vi "Station Wise_summary.vi"(0 "index":i32, 1 "Station ID":string, 3 "error in (no error)":errorcluster, 4 "Station Name":string) -> (6 "S":bool, 7 "M":bool, 9 "error out":errorcluster)   [LabVIEW 2017]
uses:
  <vilib>/addons/database/Connection.llb/DB Tools Open Connec (Path).vi
  Globle/Current date.vi
  <vilib>/addons/database/NI_Database_API.lvlib
panel:
  out "Station Name":string
  in  "Cancel Button":bool
  out "G Ack 2":bool
  out "GL 2":bool
  out "Duration P":dbl format="%<%M:%S>t"
  out "Duration Q":dbl format="%<%M:%S>t"
  out "Duration M":dbl format="%<%M:%S>t"
  out "Duration L":dbl format="%<%M:%S>t"
  out "Duration GL":dbl format="%<%M:%S>t"
  out "COUNT P":i32
  out "COUNT  Q":i32
  out "COUNT  M":i32
  out "COUNT  Mat":i32
  out "P Ack":bool
  out "Q Ack":bool
  out "M Ack":bool
  out "L Ack":bool
  out "G Ack":bool
  out "SS":bool
  out "Q":bool
  out "M":bool
  out "COUNT Safety":i32
  out "P Duration Min":dbl format="%<%M:%S>t"
  out "Q Duration Min":dbl format="%<%M:%S>t"
  out "M Duration Min":dbl format="%<%M:%S>t"
  out "L Duration Min":dbl format="%<%M:%S>t"
  out "GL Duration min":dbl format="%<%M:%S>t"
  out "P Counter":i32
  out "Q Counter":i32
  out "M Counter":i32
  out "Mat Counter":i32
  out "Safety Counter":i32
  # "Station Wise Live Breakdown Status"
  # "Safety"
  # "Material"
  # "Maintenance"
  # "Quality"
  # "Startup/Setup"
  # "Stakeholder"
  # "Count"
  # "Duration"
  # "Station"
  # "Breakdown Name"
  # "Safety"
  # "Min"
  # "Breakdown"
  # "Material"
  # "Min"
  # "Acknowledgement"
  # "Maintenance"
  # "Min"
  # "Total Count"
  # "Quality"
  # "Min"
  # "Total Duration (Min)"
  # "Startup/Setup"
  # "Min"
  # "Designed And Developed By - Infinity Automation Systems Pvt. Ltd."
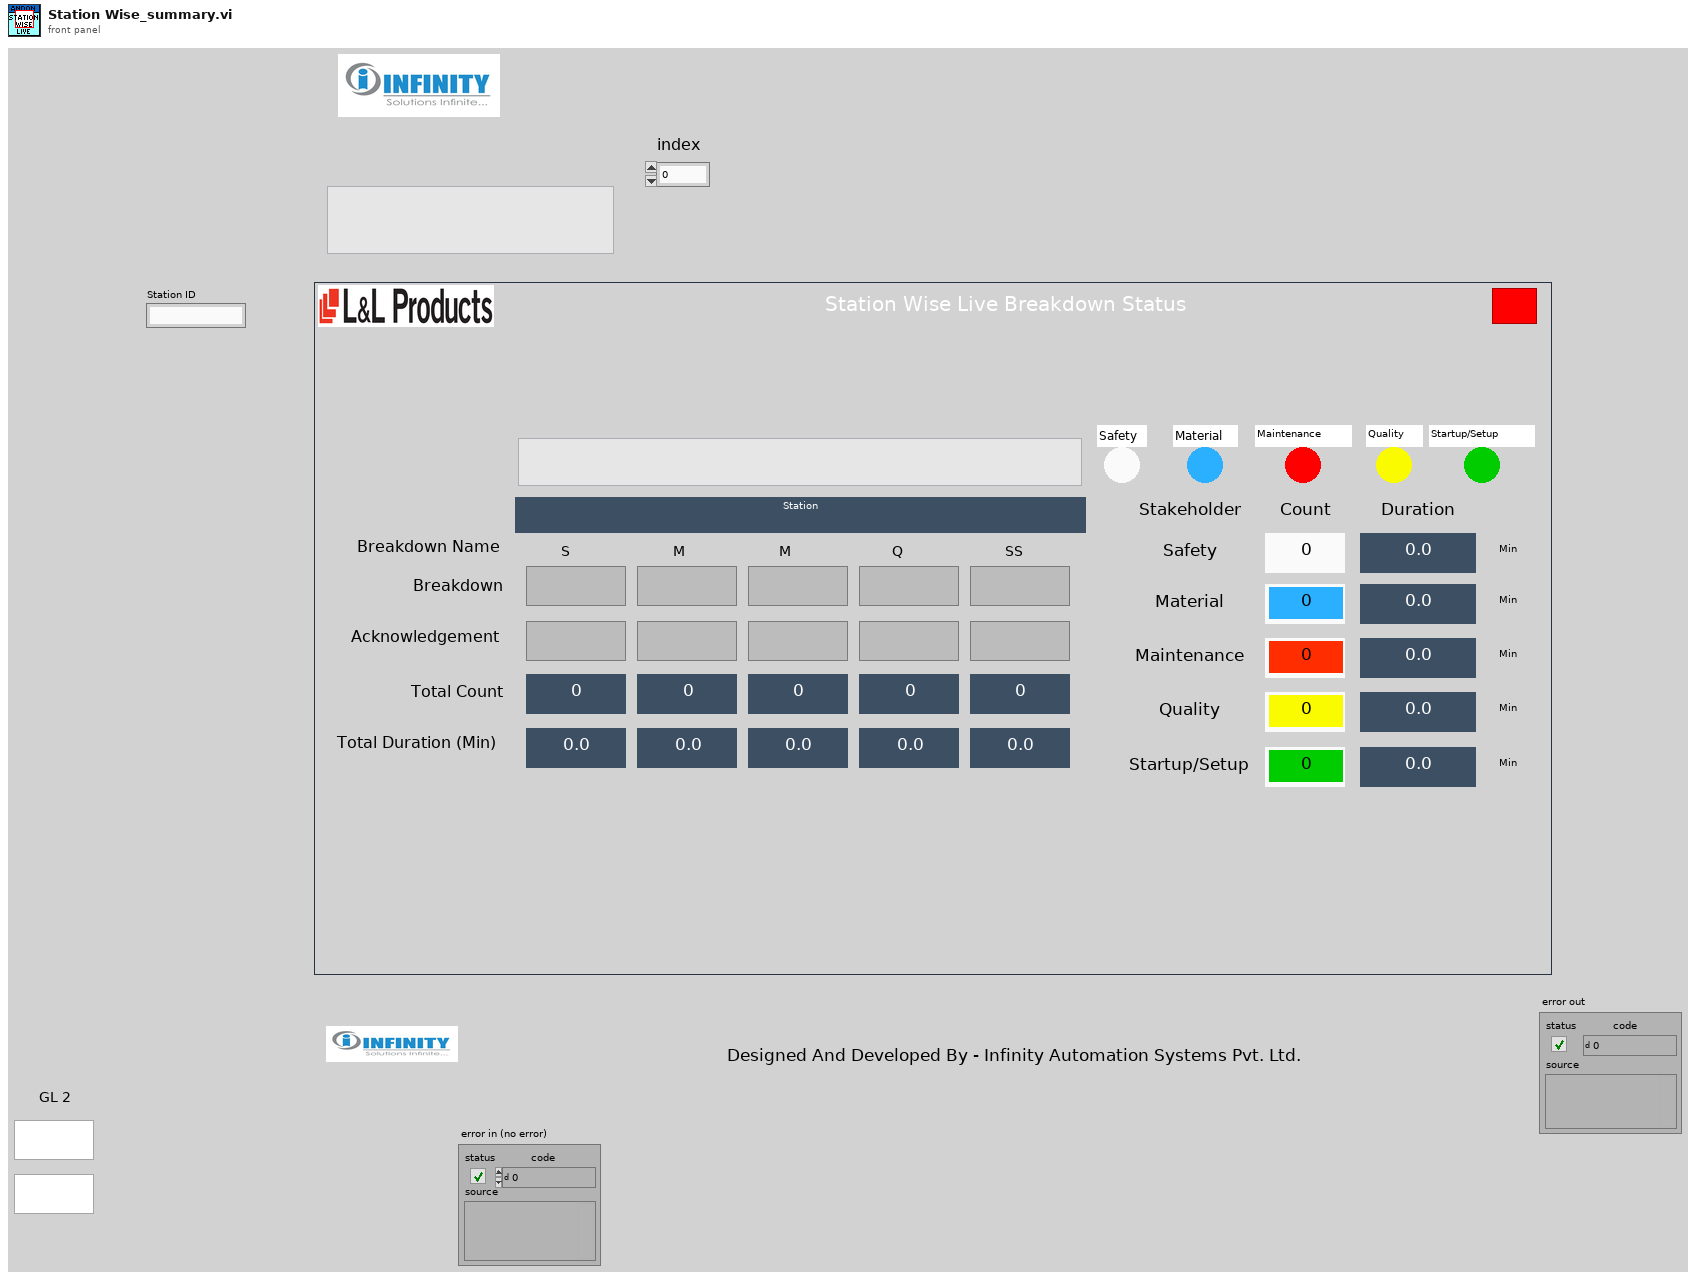
[diagram p1: front panel]
types:
  T1 = typedef "NI_Database_API.lvlib/Conn ObjectReference.ctl" = refnum<k1>
  T2 = enum32{"invalid app kind", "Development System", "Run Time System", "Student Edition", "Embedded LabVIEW", "Evaluation", "Custom"}
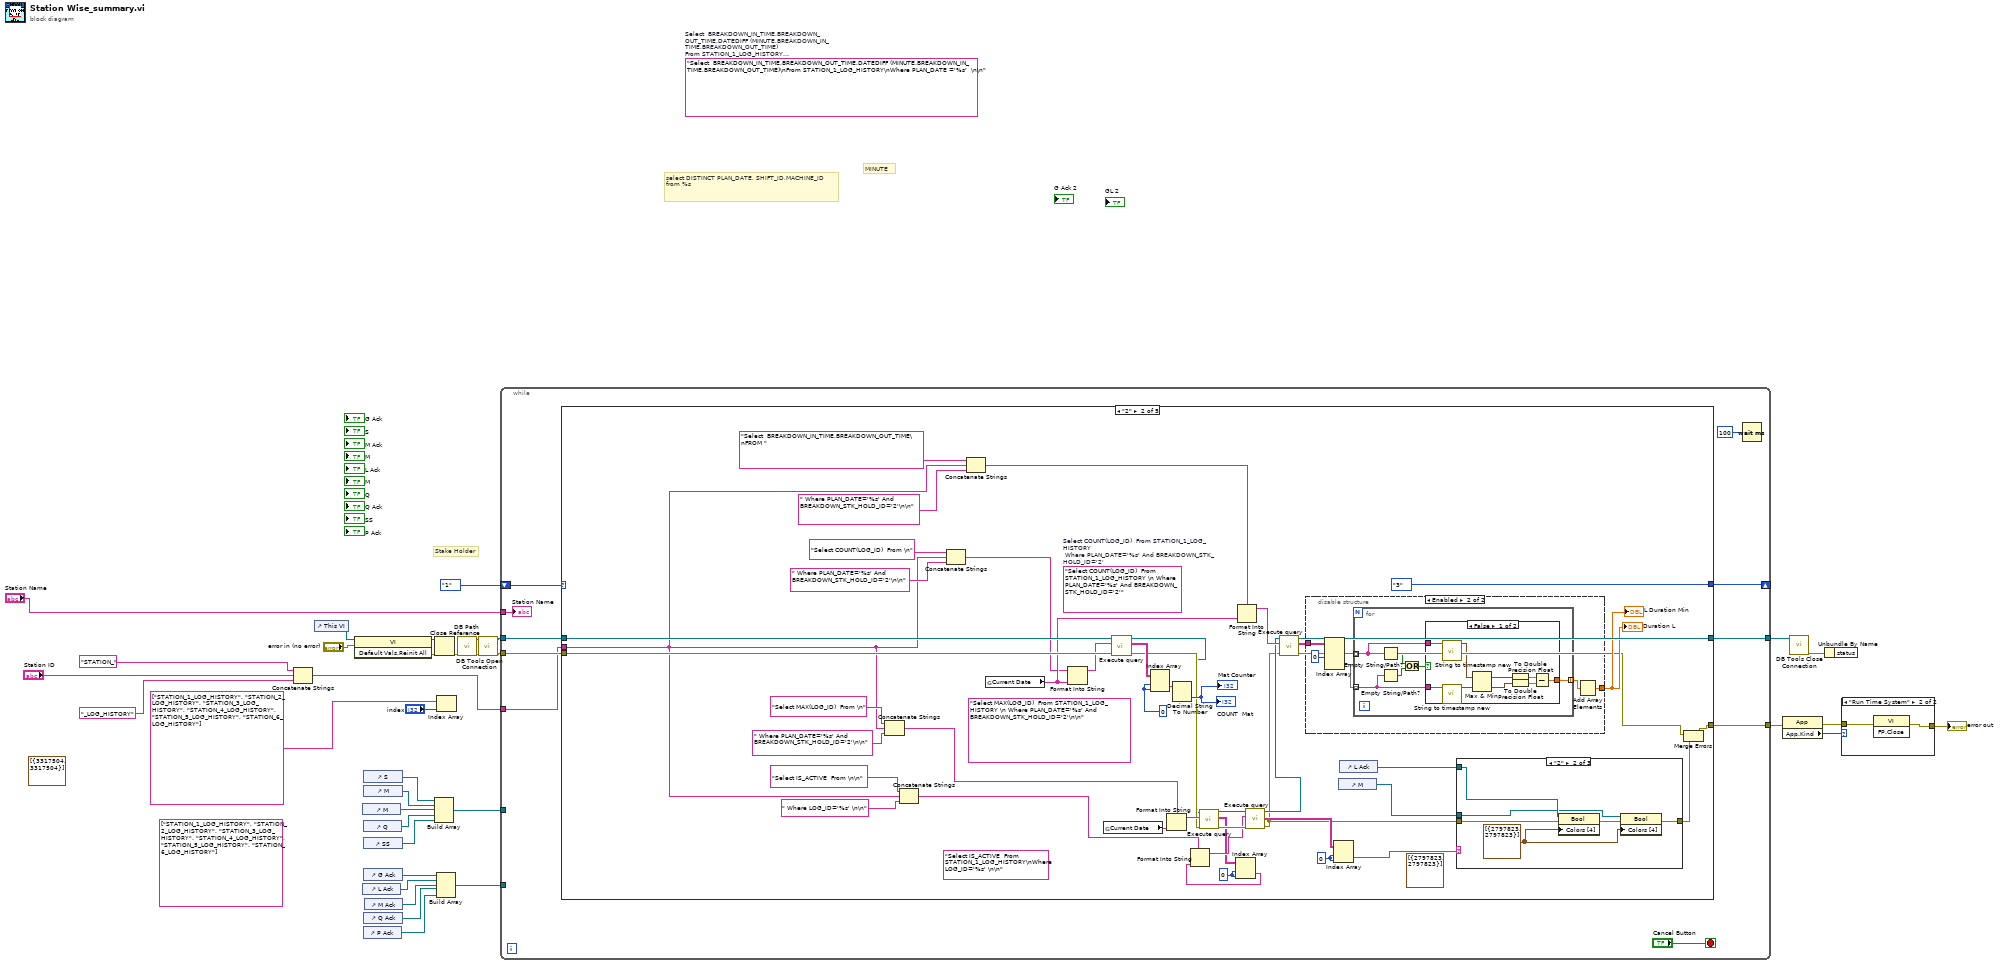
[diagram p0: block diagram]
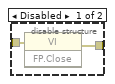
[diagram p3: hidden frame]
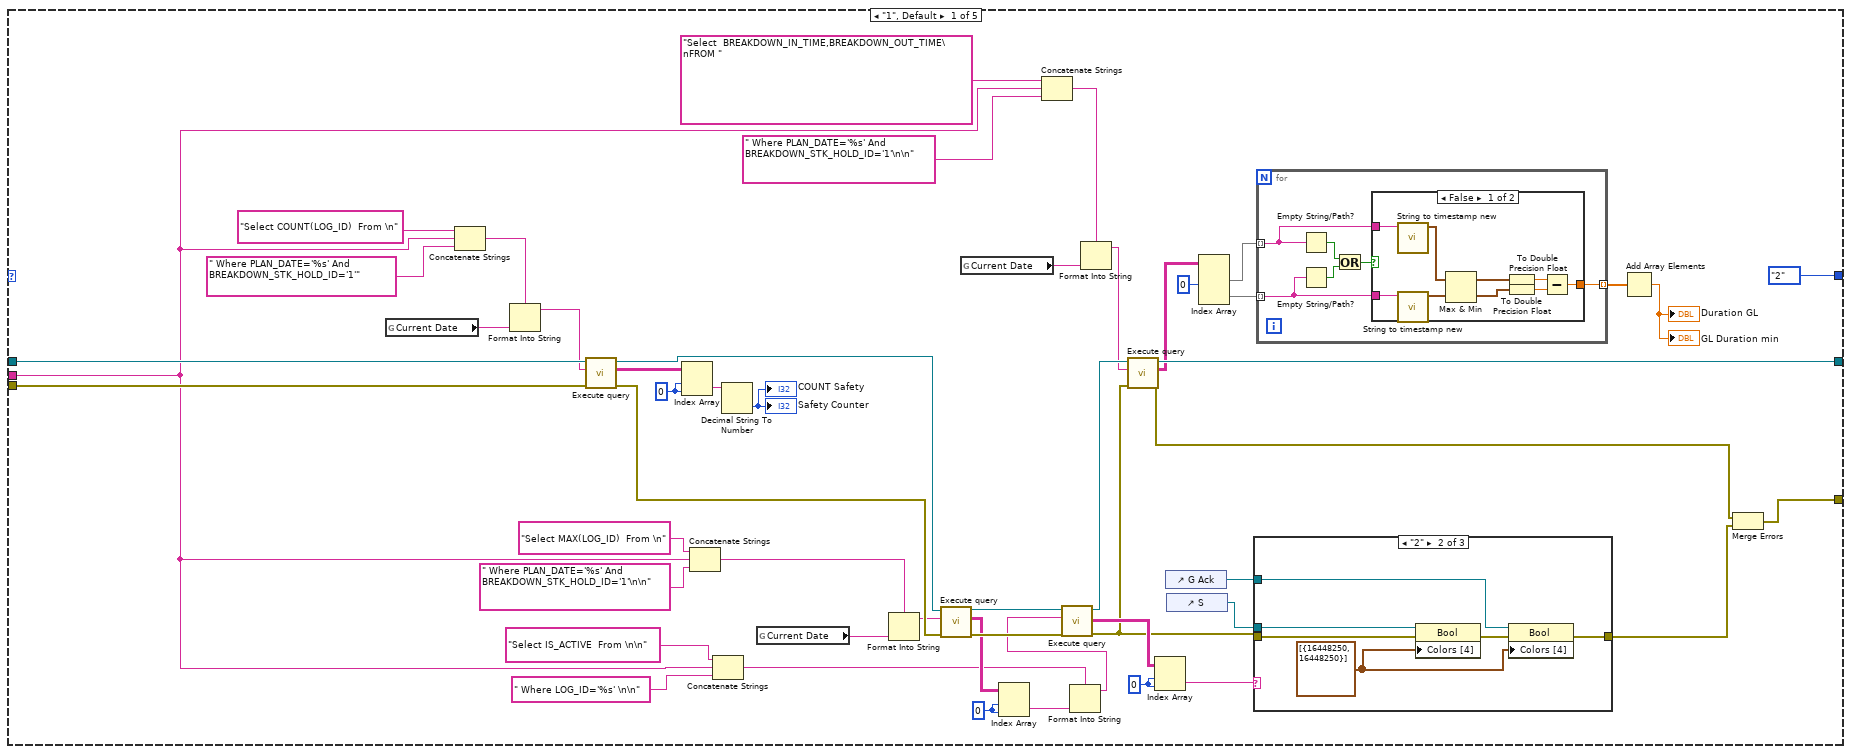
[diagram p4: hidden frame]
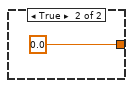
[diagram p5: hidden frame]
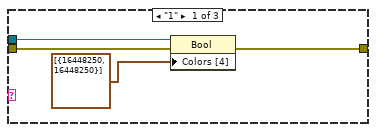
[diagram p6: hidden frame]
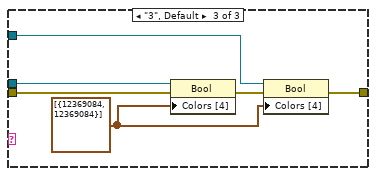
[diagram p7: hidden frame]
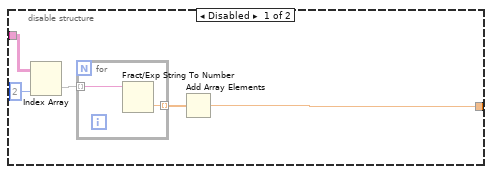
[diagram p8: hidden frame]
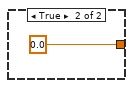
[diagram p9: hidden frame]
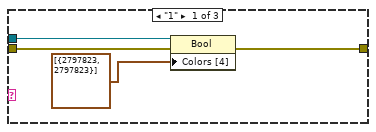
[diagram p10: hidden frame]
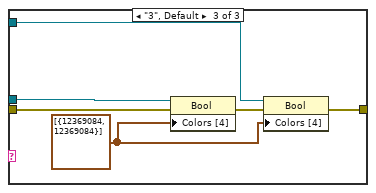
[diagram p11: hidden frame]
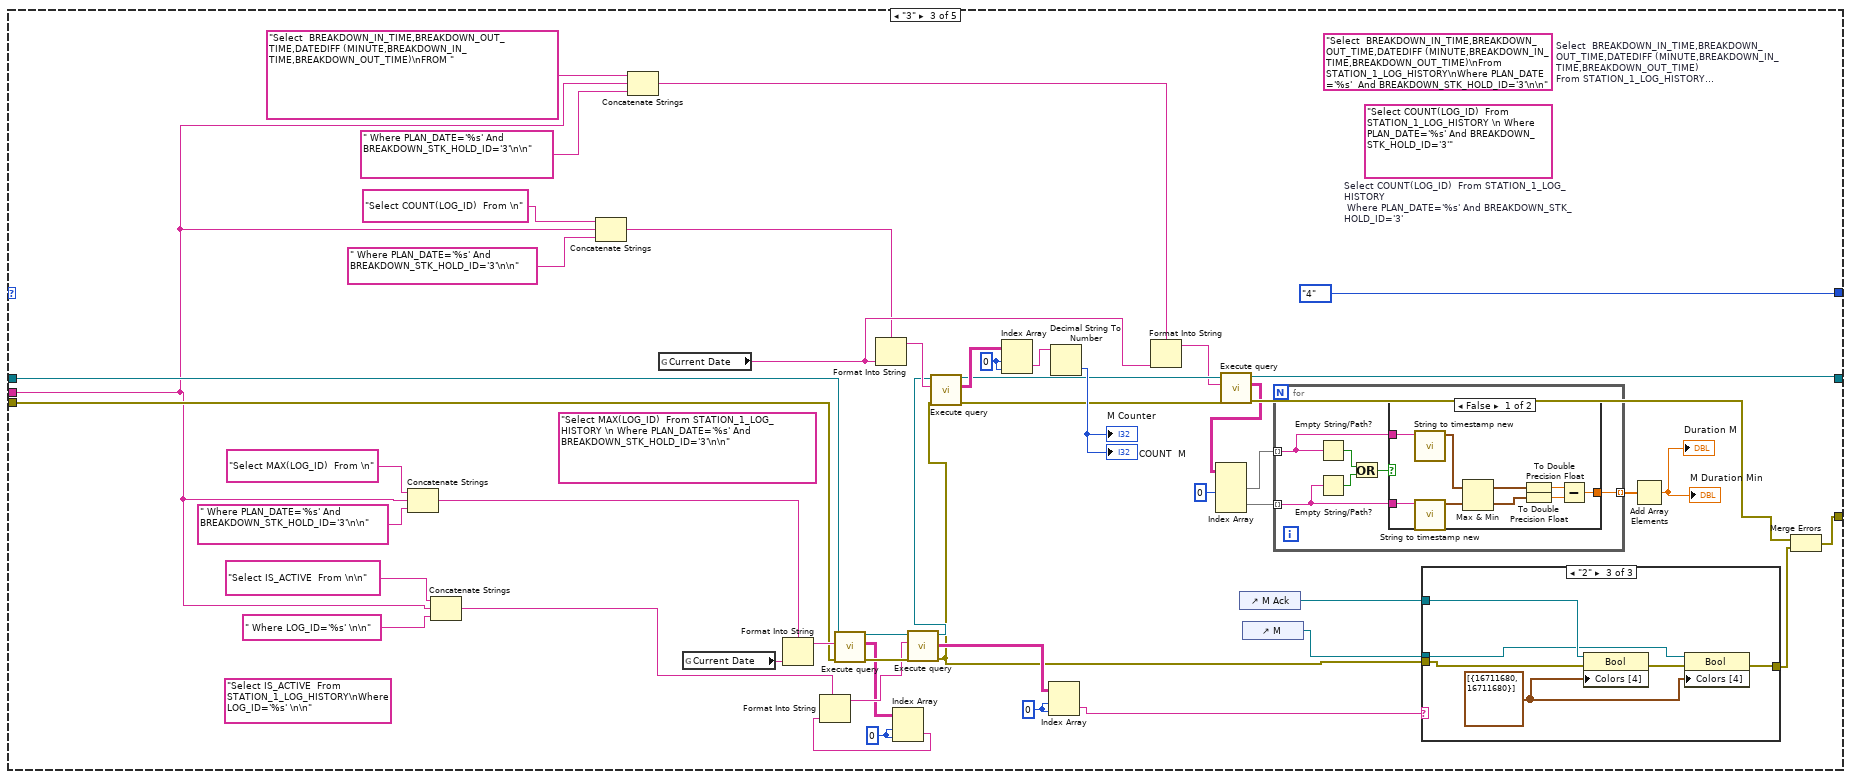
[diagram p12: hidden frame]
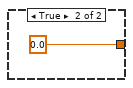
[diagram p13: hidden frame]
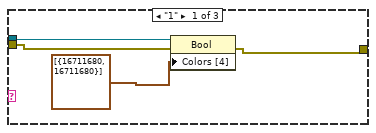
[diagram p14: hidden frame]
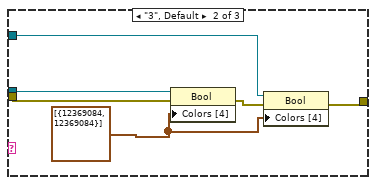
[diagram p15: hidden frame]
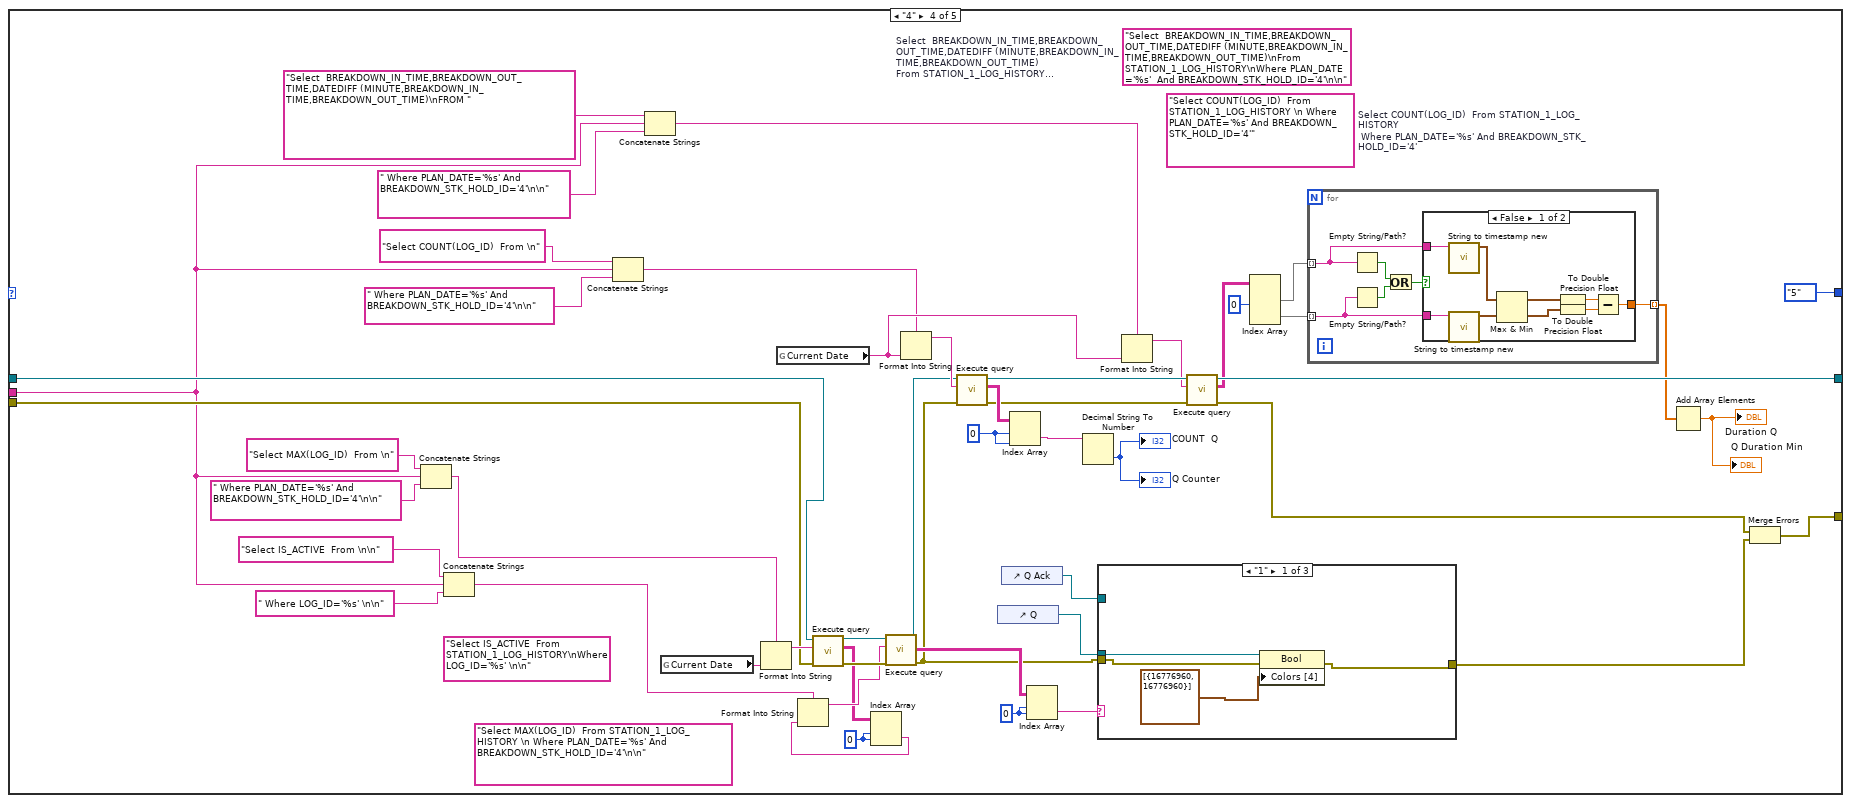
[diagram p16: hidden frame]
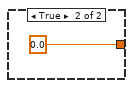
[diagram p17: hidden frame]
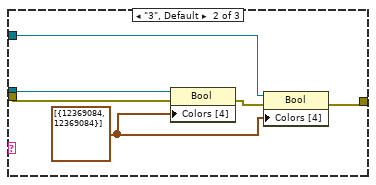
[diagram p18: hidden frame]
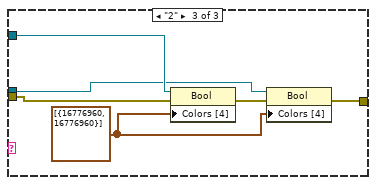
[diagram p19: hidden frame]
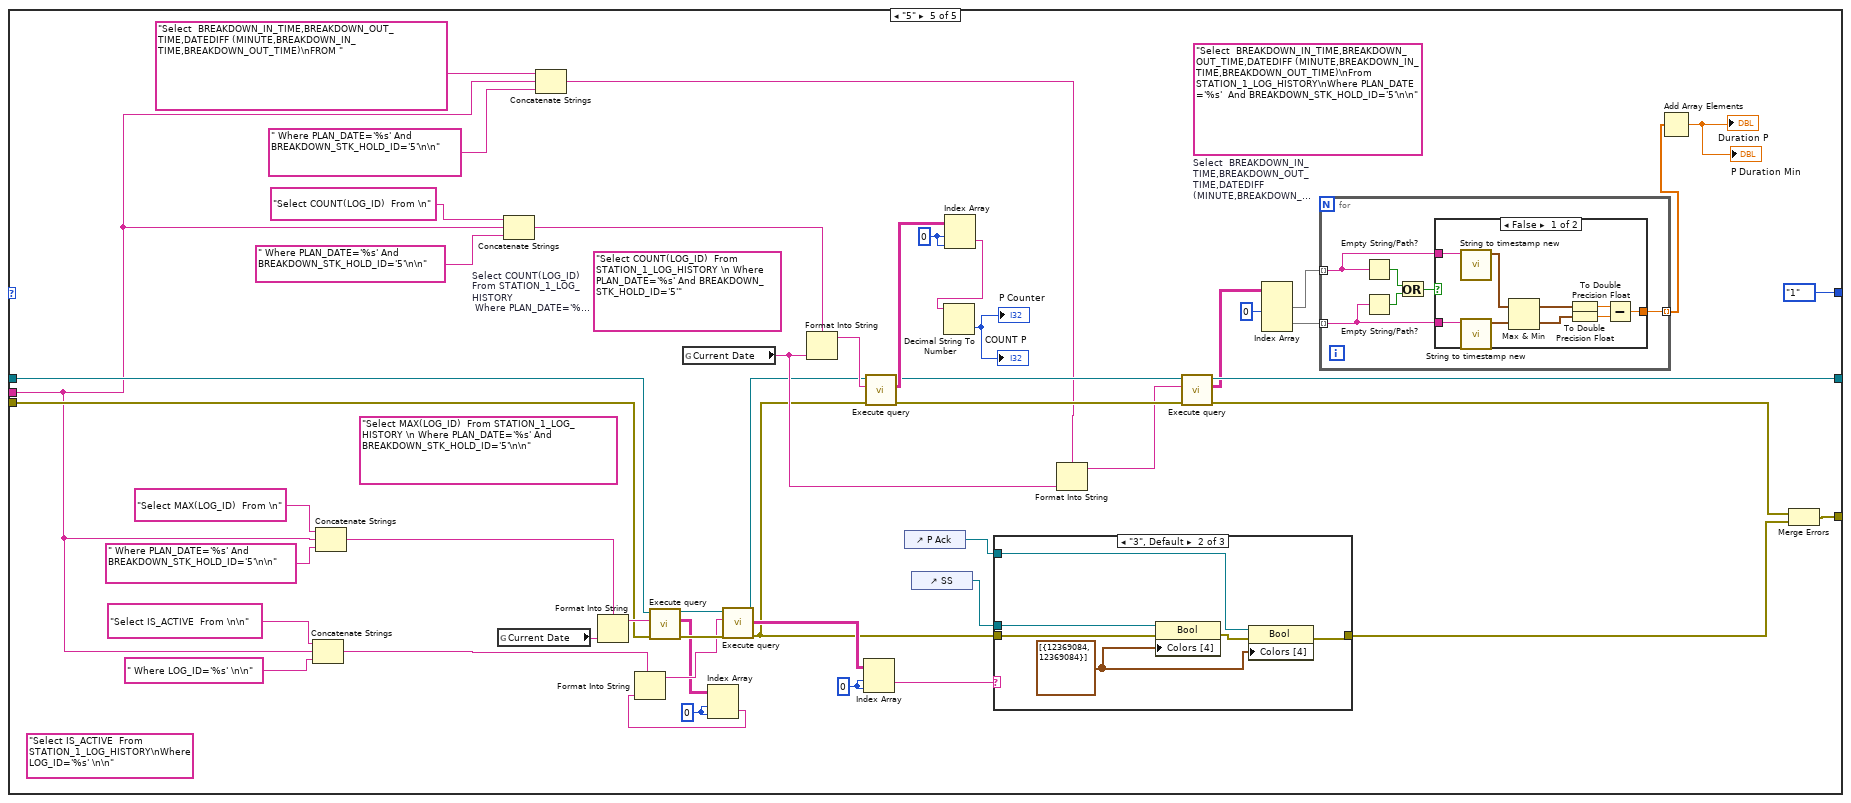
[diagram p20: hidden frame]
diagram:
  (unwired) string[] ["STATION_1_LOG_HISTORY", "STATION_2_LOG_HISTORY", "STATION_3_LOG_HISTORY", "STATION_4_LOG_HISTORY", "STATION_5_LOG_HISTORY", "STATION_6_LOG_HISTORY"]
  (unwired) "Select  BREAKDOWN_IN_TIME,BREAKDOWN_OUT_TIME,DATEDIFF (MINUTE,BREAKDOWN_IN_TIME,BREAKDOWN_OUT_TIME)\nFrom STATION_1_LOG_HISTORY\nWhere PLAN_DATE ='%s'  \n\n"  # Select  BREAKDOWN_IN_TIME,BREAKDOWN_OUT_TIME,DATEDIFF (MINUTE,BREAKDOWN_IN_TIME,BREAKDOWN_OUT_TIME) From STATION_1_LOG_HISTORY Where PLAN_DATE ='%s'
  (unwired) cluster{u32, u32}[] [{3317504, 3317504}] ("Colors [4]")
  # "Stake Holder"
  # "MINUTE"
  # "select DISTINCT PLAN_DATE, SHIFT_ID,MACHINE_ID\nfrom %s"
  n1 = Concatenate Strings("STATION_", "Station ID", "_LOG_HISTORY") -> (w5:string)
  n2 = control-ref of="This VI"() -> (w35:refnum<vi>)
  n3 = invoke class="VI" method="Default Vals.Reinit All"(reference=w35, error in="error in (no error)") -> (reference out=w33:refnum<vi>, error out=w34:errorcluster)  [unwired: 1 in, 1 out]
  n4 = control-ref of="M"() -> (w21:refnum<vi>)
  n5 = control-ref of="L Ack"() -> (w17:refnum<vi>)
  n6 = control-ref of="Q"() -> (w20:refnum<vi>)
  n7 = control-ref of="P Ack"() -> (w14:refnum<vi>)
  n8 = control-ref of="S"() -> (w23:refnum<vi>)
  n9 = control-ref of="M"() -> (w22:refnum<vi>)
  n10 = control-ref of="SS"() -> (w19:refnum<vi>)
  n11 = control-ref of="G Ack"() -> (w18:refnum<vi>)
  n12 = control-ref of="Q Ack"() -> (w15:refnum<vi>)
  n13 = control-ref of="M Ack"() -> (w16:refnum<vi>)
  n14 = Build Array(w23, w22, w21, w20, w19) -> (w13:refnum<vi>[])
  n15 = Close Reference(reference=w33, error in (no error)=w34) -> (error out=w29:errorcluster)
  n16 = Build Array(w18, w17, w16, w15, w14) -> (w12:refnum<vi>[])
  n17 = Index Array(array=string[] ["STATION_1_LOG_HISTORY", "STATION_2_LOG_HISTORY", "STATION_3_LOG_HISTORY", "STATION_4_LOG_HISTORY", "STATION_5_LOG_HISTORY", "STATION_6_LOG_HISTORY"], index="index") -> ()  [unwired: 1 out]
  n18 = call "DB Path.vi"("error in"=w29) -> ("error out"=w28:errorcluster, "DB Path"=w27:path)  [unwired: 9 in]
  n19 = call-poly <vilib>:"DB Tools Open Connection.vi"("error in (no error)"=w28, "connection information"=w27) -> ("error out"=w9:errorcluster, "connection reference"=w26:T1)  [unwired: 6 in]
  n20 = while {
    tunnel: w9 -> [w40]
    tunnel: [w45] -> w30
    tunnel: w26 -> [w41]
    tunnel: w5 -> [w39]
    shift-right: [w43] -> _
    shift-left: enum16{"1", "2", "3", "4", "5"}."1" -> [w44]
    tunnel: [w42] -> w8
    tunnel: w13 -> [_]
    tunnel: w12 -> [_]
    tunnel: "Station Name" -> [w36]
    stop <- "Cancel Button" stop-if-true
    n21 = case shown="\"2\"" w44 {
      tunnel: w40 -> [w90 w172 w244 w328 w411]
      tunnel: w41 -> [w96 w171 w243 w327 w410]
      tunnel: w39 -> [w58 w130 w226 w307 w392]
      tunnel: [w72 w145 w255 w320 w404] -> w45
      tunnel: [enum16{"1", "2", "3", "4", "5"}."2" enum16{"1", "2", "3", "4", "5"}."3" enum16{"1", "2", "3", "4", "5"}."4" enum16{"1", "2", "3", "4", "5"}."5" enum16{"1", "2", "3", "4", "5"}."1"] -> w43
      tunnel: [w91 w166 w261 w343 w425] -> w42
      frame "1", Default {
        w76 = 0 ("index (row)")
        w79 = 0 ("index (row)")
        w93 = 0 ("index (row)")
        n22 = global read "Current date.vi" "Current Date"() -> (w89:string)
        n23 = Concatenate Strings("Select COUNT(LOG_ID)  From \n", w58, " Where PLAN_DATE='%s' And BREAKDOWN_STK_HOLD_ID='1'") -> (w53:string)
        n24 = Format Into String(format string=w53, w89) -> (resulting string=w63:string)  [unwired: 2 in, 1 out]
        n25 = call "Execute query.vi"("error in (no error)"=w90, "String"=w63, "connection reference"=w96) -> ("error out"=w86:errorcluster, "Table"=w88:string[][], "connection reference 2"=w84:T1)  [unwired: 3 in, 3 out]
        n26 = Index Array(array=w88, index (row)=w93, index (col)=w93) -> (element=w92:string)
        n27 = Concatenate Strings("Select MAX(LOG_ID)  From \n", w58, " Where PLAN_DATE='%s' And BREAKDOWN_STK_HOLD_ID='1'\n\n") -> (w52:string)
        n28 = Concatenate Strings("Select IS_ACTIVE  From \n\n", w58, " Where LOG_ID='%s' \n\n") -> (w55:string)
        n29 = Decimal String To Number(string=w92) -> (number=→"Safety Counter" →"COUNT Safety":i32)  [unwired: 2 in, 1 out]
        n30 = global read "Current date.vi" "Current Date"() -> (w87:string)
        n31 = Format Into String(format string=w52, w87) -> (resulting string=w85:string)  [unwired: 2 in, 1 out]
        n32 = call "Execute query.vi"("error in (no error)"=w86, "String"=w85, "connection reference"=w84) -> ("error out"=w83:errorcluster, "Table"=w78:string[][], "connection reference 2"=w82:T1)  [unwired: 3 in, 3 out]
        n33 = global read "Current date.vi" "Current Date"() -> (w65:string)
        n34 = Index Array(array=w78, index (row)=w79, index (col)=w79) -> (element=w77:string)
        n35 = Concatenate Strings("Select  BREAKDOWN_IN_TIME,BREAKDOWN_OUT_TIME\nFROM " ("SQL query"), w58, " Where PLAN_DATE='%s' And BREAKDOWN_STK_HOLD_ID='1'\n\n") -> (w54:string)
        n36 = Format Into String(format string=w55, w77) -> (resulting string=w80:string)  [unwired: 2 in, 1 out]
        n37 = call "Execute query.vi"("error in (no error)"=w83, "String"=w80, "connection reference"=w82) -> ("error out"=w74:errorcluster, "Table"=w75:string[][], "connection reference 2"=w81:T1)  [unwired: 3 in, 3 out]
        n38 = Format Into String(format string=w54, w65) -> (resulting string=w64:string)  [unwired: 2 in, 1 out]
        n39 = call "Execute query.vi"("error in (no error)"=w74, "String"=w64, "connection reference"=w81) -> ("error out"=w73:errorcluster, "Table"=w51:string[][], "connection reference 2"=w91:T1)  [unwired: 3 in, 3 out]
        n40 = Index Array(array=w75, index (row)=w76, index (col)=w76) -> (element=w68:string)
        n41 = control-ref of="G Ack"() -> (w69:refnum<vi>)
        n42 = control-ref of="S"() -> (w70:refnum<vi>)
        n43 = Index Array(array=w51, index (col) #1=0 ("disabled index (col)")) -> (element #1=w49:string[], element #2=w48:string[])  [unwired: 3 in]
        n44 = case shown="\"2\"" w68 {
          tunnel: w74 -> [w116 w122 w128]
          tunnel: [w114 w119 w125] -> w71
          tunnel: w70 -> [w113 w118 w124]
          tunnel: w69 -> [_ w117 w123]
          frame "1" {
            n45 = property class="Bool"(reference=w113, error in=w116, "Colors [4]"=cluster{u32, u32}[] [{16448250, 16448250}]) -> (error out=w114:errorcluster)  [unwired: 1 out]
          }
          frame "2" {
            w120 = cluster{u32, u32}[] [{16448250, 16448250}] ("Colors [4]")
            n46 = property class="Bool"(reference=w118, error in=w122, "Colors [4]"=w120) -> (error out=w121:errorcluster)  [unwired: 1 out]
            n47 = property class="Bool"(reference=w117, error in=w121, "Colors [4]"=w120) -> (error out=w119:errorcluster)  [unwired: 1 out]
          }
          frame "3", Default {
            w126 = cluster{u32, u32}[] [{12369084, 12369084}] ("Colors [4]")
            n48 = property class="Bool"(reference=w124, error in=w128, "Colors [4]"=w126) -> (error out=w127:errorcluster)  [unwired: 1 out]
            n49 = property class="Bool"(reference=w123, error in=w127, "Colors [4]"=w126) -> (error out=w125:errorcluster)  [unwired: 1 out]
          }
        }
        n50 = for {
          tunnel: w49 -> [w98] mode=indexing
          tunnel: w48 -> [w99] mode=indexing
          tunnel: [w97] -> w47 mode=indexing
          n51 = Empty String/Path?(string/path=w98) -> (empty?=w101:bool)
          n52 = Empty String/Path?(string/path=w99) -> (empty?=w102:bool)
          n53 = Or(x=w101, y=w102) -> (x .or. y?=w100:bool)
          n54 = case shown="False" w100 {
            tunnel: [w105 0.0] -> w97
            tunnel: w98 -> [w104 _]
            tunnel: w99 -> [w103 _]
            frame False {
              n55 = call "String to timestamp new.vi"("String Timestamp"=w104) -> ("Timestamp"=w107:timestamp)  [unwired: 10 in]
              n56 = call "String to timestamp new.vi"("String Timestamp"=w103) -> ("Timestamp"=w106:timestamp)  [unwired: 10 in]
              n57 = Max & Min(x=w107, y=w106) -> (max(x,y)=w111:timestamp, min(x,y)=w110:timestamp)
              n58 = To Double Precision Float(number=w111) -> (double precision float=w109:dbl)
              n59 = To Double Precision Float(number=w110) -> (double precision float=w108:dbl)
              n60 = Subtract(x=w109, y=w108) -> (x-y=w105:dbl)
            }
            frame True {
            }
          }
        }
        n61 = Add Array Elements(numeric array=w47) -> (sum=→"GL Duration min" →"Duration GL":dbl)
        n62 = Merge Errors(w73, w71) -> (w72:errorcluster)
      }
      frame "2" {
        (unwired) cluster{u32, u32}[] [{2797823, 2797823}] ("Colors [4]")
        w154 = 0 ("index (row)")
        w157 = 0 ("index (row)")
        (unwired) "Select IS_ACTIVE  From STATION_1_LOG_HISTORY\nWhere LOG_ID='%s' \n\n"
        (unwired) "Select MAX(LOG_ID)  From STATION_1_LOG_HISTORY \n Where PLAN_DATE='%s' And BREAKDOWN_STK_HOLD_ID='2'\n\n"
        w168 = 0 ("index (row)")
        (unwired) "Select COUNT(LOG_ID)  From STATION_1_LOG_HISTORY \n Where PLAN_DATE='%s' And BREAKDOWN_STK_HOLD_ID='2'"  # Select COUNT(LOG_ID)  From STATION_1_LOG_HISTORY   Where PLAN_DATE='%s' And BREAKDOWN_STK_HOLD_ID='2'
        n63 = Concatenate Strings("Select MAX(LOG_ID)  From \n", w130, " Where PLAN_DATE='%s' And BREAKDOWN_STK_HOLD_ID='2'\n\n") -> (w132:string)
        n64 = Concatenate Strings("Select IS_ACTIVE  From \n\n", w130, " Where LOG_ID='%s' \n\n") -> (w131:string)
        n65 = Concatenate Strings("Select COUNT(LOG_ID)  From \n", w130, " Where PLAN_DATE='%s' And BREAKDOWN_STK_HOLD_ID='2'\n\n") -> (w137:string)
        n66 = Concatenate Strings("Select  BREAKDOWN_IN_TIME,BREAKDOWN_OUT_TIME\nFROM " ("SQL query"), w130, " Where PLAN_DATE='%s' And BREAKDOWN_STK_HOLD_ID='2'\n\n") -> (w140:string)
        n67 = global read "Current date.vi" "Current Date"() -> (w165:string)
        n68 = Format Into String(format string=w137, w165) -> (resulting string=w170:string)  [unwired: 2 in, 1 out]
        n69 = global read "Current date.vi" "Current Date"() -> (w162:string)
        n70 = call "Execute query.vi"("error in (no error)"=w172, "String"=w170, "connection reference"=w171) -> ("error out"=w152:errorcluster, "Table"=w169:string[][], "connection reference 2"=w150:T1)  [unwired: 3 in, 3 out]
        n71 = Index Array(array=w169, index (row)=w168, index (col)=w168) -> (element=w167:string)
        n72 = Format Into String(format string=w132, w162) -> (resulting string=w161:string)  [unwired: 2 in, 1 out]
        n73 = Decimal String To Number(string=w167) -> (number=→"Mat Counter" →"COUNT  Mat":i32)  [unwired: 2 in, 1 out]
        n74 = call "Execute query.vi"("error in (no error)"=w152, "String"=w161, "connection reference"=w150) -> ("error out"=w160:errorcluster, "Table"=w156:string[][], "connection reference 2"=w159:T1)  [unwired: 3 in, 3 out]
        n75 = Index Array(array=w156, index (row)=w157, index (col)=w157) -> (element=w155:string)
        n76 = Format Into String(format string=w131, w155) -> (resulting string=w158:string)  [unwired: 2 in, 1 out]
        n77 = Format Into String(format string=w140, w165) -> (resulting string=w164:string)  [unwired: 2 in, 1 out]
        n78 = call "Execute query.vi"("error in (no error)"=w160, "String"=w158, "connection reference"=w159) -> ("error out"=w148:errorcluster, "Table"=w153:string[][], "connection reference 2"=w151:T1)  [unwired: 3 in, 3 out]
        n79 = call "Execute query.vi"("error in (no error)"=w148, "String"=w164, "connection reference"=w151) -> ("error out"=w146:errorcluster, "Table"=w129:string[][], "connection reference 2"=w166:T1)  [unwired: 3 in, 3 out]
        n80 = disable-structure shown="Enabled" {
          disable-tunnel: [w176 w183] -> w163
          disable-tunnel: w129 -> [w175 w187]
          frame Disabled {
            n81 = Index Array(array=w175, index (col)=2 ("disabled index (col)")) -> (element=w177:string[])  [unwired: 1 in]
            n82 = for {
              tunnel: w177 -> [w181] mode=indexing
              tunnel: [w180] -> w179 mode=indexing
              n83 = Fract/Exp String To Number(string=w181) -> (number=w180:dbl)  [unwired: 3 in, 1 out]
            }
            n84 = Add Array Elements(numeric array=w179) -> (sum=w176:dbl)
          }
          frame Enabled {
            n85 = Index Array(array=w187, index (col) #1=0 ("disabled index (col)")) -> (element #1=w185:string[], element #2=w184:string[])  [unwired: 3 in]
            n86 = for {
              tunnel: w185 -> [w189] mode=indexing
              tunnel: w184 -> [w190] mode=indexing
              tunnel: [w188] -> w182 mode=indexing
              n87 = Empty String/Path?(string/path=w189) -> (empty?=w192:bool)
              n88 = Empty String/Path?(string/path=w190) -> (empty?=w193:bool)
              n89 = Or(x=w192, y=w193) -> (x .or. y?=w191:bool)
              n90 = case shown="False" w191 {
                tunnel: [w196 0.0] -> w188
                tunnel: w189 -> [w195 _]
                tunnel: w190 -> [w194 _]
                frame False {
                  n91 = call "String to timestamp new.vi"("String Timestamp"=w195) -> ("Timestamp"=w198:timestamp)  [unwired: 10 in]
                  n92 = call "String to timestamp new.vi"("String Timestamp"=w194) -> ("Timestamp"=w197:timestamp)  [unwired: 10 in]
                  n93 = Max & Min(x=w198, y=w197) -> (max(x,y)=w202:timestamp, min(x,y)=w201:timestamp)
                  n94 = To Double Precision Float(number=w202) -> (double precision float=w200:dbl)
                  n95 = To Double Precision Float(number=w201) -> (double precision float=w199:dbl)
                  n96 = Subtract(x=w200, y=w199) -> (x-y=w196:dbl)
                }
                frame True {
                }
              }
            }
            n97 = Add Array Elements(numeric array=w182) -> (sum=w183:dbl)
          }
        }
        "L Duration Min" <- w163
        "Duration L" <- w163
        n98 = Index Array(array=w153, index (row)=w154, index (col)=w154) -> (element=w149:string)
        n99 = control-ref of="M"() -> (w144:refnum<vi>)
        n100 = control-ref of="L Ack"() -> (w143:refnum<vi>)
        n101 = case shown="\"2\"" w149 {
          tunnel: w148 -> [w207 w213 w219]
          tunnel: [w204 w209 w216] -> w147
          tunnel: w144 -> [w205 w211 w215]
          tunnel: w143 -> [_ w212 w214]
          frame "1" {
            n102 = property class="Bool"(reference=w205, error in=w207, "Colors [4]"=cluster{u32, u32}[] [{2797823, 2797823}]) -> (error out=w204:errorcluster)  [unwired: 1 out]
          }
          frame "2" {
            w208 = cluster{u32, u32}[] [{2797823, 2797823}] ("Colors [4]")
            n103 = property class="Bool"(reference=w212, error in=w213, "Colors [4]"=w208) -> (error out=w210:errorcluster)  [unwired: 1 out]
            n104 = property class="Bool"(reference=w211, error in=w210, "Colors [4]"=w208) -> (error out=w209:errorcluster)  [unwired: 1 out]
          }
          frame "3", Default {
            w217 = cluster{u32, u32}[] [{12369084, 12369084}] ("Colors [4]")
            n105 = property class="Bool"(reference=w215, error in=w219, "Colors [4]"=w217) -> (error out=w218:errorcluster)  [unwired: 1 out]
            n106 = property class="Bool"(reference=w214, error in=w218, "Colors [4]"=w217) -> (error out=w216:errorcluster)  [unwired: 1 out]
          }
        }
        n107 = Merge Errors(w146, w147) -> (w145:errorcluster)
      }
      frame "3" {
        w246 = 0 ("index (row)")
        w249 = 0 ("index (row)")
        (unwired) "Select IS_ACTIVE  From STATION_1_LOG_HISTORY\nWhere LOG_ID='%s' \n\n"
        (unwired) "Select MAX(LOG_ID)  From STATION_1_LOG_HISTORY \n Where PLAN_DATE='%s' And BREAKDOWN_STK_HOLD_ID='3'\n\n"
        (unwired) "Select  BREAKDOWN_IN_TIME,BREAKDOWN_OUT_TIME,DATEDIFF (MINUTE,BREAKDOWN_IN_TIME,BREAKDOWN_OUT_TIME)\nFrom STATION_1_LOG_HISTORY\nWhere PLAN_DATE ='%s'  And BREAKDOWN_STK_HOLD_ID='3'\n\n"  # Select  BREAKDOWN_IN_TIME,BREAKDOWN_OUT_TIME,DATEDIFF (MINUTE,BREAKDOWN_IN_TIME,BREAKDOWN_OUT_TIME) From STATION_1_LOG_HISTORY Where PLAN_DATE ='%s'  And BREAKDOWN_STK_HOLD_ID='3'
        w265 = 0 ("index (row)")
        (unwired) "Select COUNT(LOG_ID)  From STATION_1_LOG_HISTORY \n Where PLAN_DATE='%s' And BREAKDOWN_STK_HOLD_ID='3'"  # Select COUNT(LOG_ID)  From STATION_1_LOG_HISTORY   Where PLAN_DATE='%s' And BREAKDOWN_STK_HOLD_ID='3'
        n108 = Concatenate Strings("Select MAX(LOG_ID)  From \n", w226, " Where PLAN_DATE='%s' And BREAKDOWN_STK_HOLD_ID='3'\n\n") -> (w227:string)
        n109 = Concatenate Strings("Select IS_ACTIVE  From \n\n", w226, " Where LOG_ID='%s' \n\n") -> (w225:string)
        n110 = Concatenate Strings("Select COUNT(LOG_ID)  From \n", w226, " Where PLAN_DATE='%s' And BREAKDOWN_STK_HOLD_ID='3'\n\n") -> (w232:string)
        n111 = Concatenate Strings("Select  BREAKDOWN_IN_TIME,BREAKDOWN_OUT_TIME,DATEDIFF (MINUTE,BREAKDOWN_IN_TIME,BREAKDOWN_OUT_TIME)\nFROM " ("SQL query"), w226, " Where PLAN_DATE='%s' And BREAKDOWN_STK_HOLD_ID='3'\n\n") -> (w233:string)
        n112 = global read "Current date.vi" "Current Date"() -> (w260:string)
        n113 = global read "Current date.vi" "Current Date"() -> (w254:string)
        n114 = Format Into String(format string=w227, w254) -> (resulting string=w253:string)  [unwired: 2 in, 1 out]
        n115 = call "Execute query.vi"("error in (no error)"=w244, "String"=w253, "connection reference"=w243) -> ("error out"=w252:errorcluster, "Table"=w248:string[][], "connection reference 2"=w251:T1)  [unwired: 3 in, 3 out]
        n116 = Format Into String(format string=w232, w260) -> (resulting string=w267:string)  [unwired: 2 in, 1 out]
        n117 = Index Array(array=w248, index (row)=w249, index (col)=w249) -> (element=w247:string)
        n118 = Format Into String(format string=w225, w247) -> (resulting string=w250:string)  [unwired: 2 in, 1 out]
        n119 = call "Execute query.vi"("error in (no error)"=w252, "String"=w250, "connection reference"=w251) -> ("error out"=w238:errorcluster, "Table"=w245:string[][], "connection reference 2"=w242:T1)  [unwired: 3 in, 3 out]
        n120 = call "Execute query.vi"("error in (no error)"=w238, "String"=w267, "connection reference"=w242) -> ("error out"=w263:errorcluster, "Table"=w266:string[][], "connection reference 2"=w262:T1)  [unwired: 3 in, 3 out]
        n121 = Index Array(array=w266, index (row)=w265, index (col)=w265) -> (element=w264:string)
        n122 = Index Array(array=w245, index (row)=w246, index (col)=w246) -> (element=w241:string)
        n123 = Decimal String To Number(string=w264) -> (number=→"M Counter" →"COUNT  M":i32)  [unwired: 2 in, 1 out]
        n124 = Format Into String(format string=w233, w260) -> (resulting string=w259:string)  [unwired: 2 in, 1 out]
        n125 = call "Execute query.vi"("error in (no error)"=w263, "String"=w259, "connection reference"=w262) -> ("error out"=w256:errorcluster, "Table"=w220:string[][], "connection reference 2"=w261:T1)  [unwired: 3 in, 3 out]
        n126 = Index Array(array=w220, index (col) #1=0 ("disabled index (col)")) -> (element #1=w223:string[], element #2=w222:string[])  [unwired: 3 in]
        n127 = control-ref of="M Ack"() -> (w240:refnum<vi>)
        n128 = control-ref of="M"() -> (w239:refnum<vi>)
        n129 = for {
          tunnel: w223 -> [w271] mode=indexing
          tunnel: w222 -> [w272] mode=indexing
          tunnel: [w270] -> w221 mode=indexing
          n130 = Empty String/Path?(string/path=w271) -> (empty?=w274:bool)
          n131 = Empty String/Path?(string/path=w272) -> (empty?=w275:bool)
          n132 = Or(x=w274, y=w275) -> (x .or. y?=w273:bool)
          n133 = case shown="False" w273 {
            tunnel: [w278 0.0] -> w270
            tunnel: w271 -> [w277 _]
            tunnel: w272 -> [w276 _]
            frame False {
              n134 = call "String to timestamp new.vi"("String Timestamp"=w277) -> ("Timestamp"=w280:timestamp)  [unwired: 10 in]
              n135 = call "String to timestamp new.vi"("String Timestamp"=w276) -> ("Timestamp"=w279:timestamp)  [unwired: 10 in]
              n136 = Max & Min(x=w280, y=w279) -> (max(x,y)=w284:timestamp, min(x,y)=w283:timestamp)
              n137 = To Double Precision Float(number=w284) -> (double precision float=w282:dbl)
              n138 = To Double Precision Float(number=w283) -> (double precision float=w281:dbl)
              n139 = Subtract(x=w282, y=w281) -> (x-y=w278:dbl)
            }
            frame True {
            }
          }
        }
        n140 = case shown="\"2\"" w241 {
          tunnel: [w286 w293 w298] -> w257
          tunnel: w240 -> [_ w292 w300]
          tunnel: w239 -> [w287 w291 w297]
          tunnel: w238 -> [w288 w290 w301]
          frame "1" {
            n141 = property class="Bool"(reference=w287, error in=w288, "Colors [4]"=cluster{u32, u32}[] [{16711680, 16711680}]) -> (error out=w286:errorcluster)  [unwired: 1 out]
          }
          frame "3", Default {
            w294 = cluster{u32, u32}[] [{12369084, 12369084}] ("Colors [4]")
            n142 = property class="Bool"(reference=w291, error in=w290, "Colors [4]"=w294) -> (error out=w295:errorcluster)  [unwired: 1 out]
            n143 = property class="Bool"(reference=w292, error in=w295, "Colors [4]"=w294) -> (error out=w293:errorcluster)  [unwired: 1 out]
          }
          frame "2" {
            w296 = cluster{u32, u32}[] [{16711680, 16711680}] ("Colors [4]")
            n144 = property class="Bool"(reference=w300, error in=w301, "Colors [4]"=w296) -> (error out=w299:errorcluster)  [unwired: 1 out]
            n145 = property class="Bool"(reference=w297, error in=w299, "Colors [4]"=w296) -> (error out=w298:errorcluster)  [unwired: 1 out]
          }
        }
        n146 = Add Array Elements(numeric array=w221) -> (sum=→"M Duration Min" →"Duration M":dbl)
        n147 = Merge Errors(w256, w257) -> (w255:errorcluster)
      }
      frame "4" {
        w330 = 0 ("index (row)")
        w329 = 0 ("index (row)")
        (unwired) "Select IS_ACTIVE  From STATION_1_LOG_HISTORY\nWhere LOG_ID='%s' \n\n"
        (unwired) "Select MAX(LOG_ID)  From STATION_1_LOG_HISTORY \n Where PLAN_DATE='%s' And BREAKDOWN_STK_HOLD_ID='4'\n\n"
        (unwired) "Select  BREAKDOWN_IN_TIME,BREAKDOWN_OUT_TIME,DATEDIFF (MINUTE,BREAKDOWN_IN_TIME,BREAKDOWN_OUT_TIME)\nFrom STATION_1_LOG_HISTORY\nWhere PLAN_DATE ='%s'  And BREAKDOWN_STK_HOLD_ID='4'\n\n"  # Select  BREAKDOWN_IN_TIME,BREAKDOWN_OUT_TIME,DATEDIFF (MINUTE,BREAKDOWN_IN_TIME,BREAKDOWN_OUT_TIME) From STATION_1_LOG_HISTORY Where PLAN_DATE ='%s'  And BREAKDOWN_STK_HOLD_ID='4'
        w347 = 0 ("index (row)")
        (unwired) "Select COUNT(LOG_ID)  From STATION_1_LOG_HISTORY \n Where PLAN_DATE='%s' And BREAKDOWN_STK_HOLD_ID='4'"  # Select COUNT(LOG_ID)  From STATION_1_LOG_HISTORY   Where PLAN_DATE='%s' And BREAKDOWN_STK_HOLD_ID='4'
        n148 = Concatenate Strings("Select MAX(LOG_ID)  From \n", w307, " Where PLAN_DATE='%s' And BREAKDOWN_STK_HOLD_ID='4'\n\n") -> (w309:string)
        n149 = Concatenate Strings("Select IS_ACTIVE  From \n\n", w307, " Where LOG_ID='%s' \n\n") -> (w308:string)
        n150 = Concatenate Strings("Select COUNT(LOG_ID)  From \n", w307, " Where PLAN_DATE='%s' And BREAKDOWN_STK_HOLD_ID='4'\n\n") -> (w314:string)
        n151 = Concatenate Strings("Select  BREAKDOWN_IN_TIME,BREAKDOWN_OUT_TIME,DATEDIFF (MINUTE,BREAKDOWN_IN_TIME,BREAKDOWN_OUT_TIME)\nFROM " ("SQL query"), w307, " Where PLAN_DATE='%s' And BREAKDOWN_STK_HOLD_ID='4'\n\n") -> (w315:string)
        n152 = global read "Current date.vi" "Current Date"() -> (w338:string)
        n153 = Format Into String(format string=w309, w338) -> (resulting string=w337:string)  [unwired: 2 in, 1 out]
        n154 = global read "Current date.vi" "Current Date"() -> (w342:string)
        n155 = call "Execute query.vi"("error in (no error)"=w328, "String"=w337, "connection reference"=w327) -> ("error out"=w336:errorcluster, "Table"=w333:string[][], "connection reference 2"=w335:T1)  [unwired: 3 in, 3 out]
        n156 = Index Array(array=w333, index (row)=w329, index (col)=w329) -> (element=w332:string)
        n157 = Format Into String(format string=w308, w332) -> (resulting string=w334:string)  [unwired: 2 in, 1 out]
        n158 = call "Execute query.vi"("error in (no error)"=w336, "String"=w334, "connection reference"=w335) -> ("error out"=w325:errorcluster, "Table"=w331:string[][], "connection reference 2"=w326:T1)  [unwired: 3 in, 3 out]
        n159 = Format Into String(format string=w314, w342) -> (resulting string=w349:string)  [unwired: 2 in, 1 out]
        n160 = call "Execute query.vi"("error in (no error)"=w325, "String"=w349, "connection reference"=w326) -> ("error out"=w345:errorcluster, "Table"=w348:string[][], "connection reference 2"=w344:T1)  [unwired: 3 in, 3 out]
        n161 = control-ref of="Q"() -> (w324:refnum<vi>)
        n162 = control-ref of="Q Ack"() -> (w323:refnum<vi>)
        n163 = Index Array(array=w348, index (row)=w347, index (col)=w347) -> (element=w346:string)
        n164 = Index Array(array=w331, index (row)=w330, index (col)=w330) -> (element=w339:string)
        n165 = Decimal String To Number(string=w346) -> (number=→"Q Counter" →"COUNT  Q":i32)  [unwired: 2 in, 1 out]
        n166 = case shown="\"1\"" w339 {
          tunnel: [w368 w375 w381] -> w321
          tunnel: w323 -> [_ w374 w382]
          tunnel: w324 -> [w369 w373 w379]
          tunnel: w325 -> [w370 w372 w383]
          frame "1" {
            n167 = property class="Bool"(reference=w369, error in=w370, "Colors [4]"=cluster{u32, u32}[] [{16776960, 16776960}]) -> (error out=w368:errorcluster)  [unwired: 1 out]
          }
          frame "3", Default {
            w376 = cluster{u32, u32}[] [{12369084, 12369084}] ("Colors [4]")
            n168 = property class="Bool"(reference=w373, error in=w372, "Colors [4]"=w376) -> (error out=w377:errorcluster)  [unwired: 1 out]
            n169 = property class="Bool"(reference=w374, error in=w377, "Colors [4]"=w376) -> (error out=w375:errorcluster)  [unwired: 1 out]
          }
          frame "2" {
            w378 = cluster{u32, u32}[] [{16776960, 16776960}] ("Colors [4]")
            n170 = property class="Bool"(reference=w382, error in=w383, "Colors [4]"=w378) -> (error out=w380:errorcluster)  [unwired: 1 out]
            n171 = property class="Bool"(reference=w379, error in=w380, "Colors [4]"=w378) -> (error out=w381:errorcluster)  [unwired: 1 out]
          }
        }
        n172 = Format Into String(format string=w315, w342) -> (resulting string=w341:string)  [unwired: 2 in, 1 out]
        n173 = call "Execute query.vi"("error in (no error)"=w345, "String"=w341, "connection reference"=w344) -> ("error out"=w322:errorcluster, "Table"=w303:string[][], "connection reference 2"=w343:T1)  [unwired: 3 in, 3 out]
        n174 = Index Array(array=w303, index (col) #1=0 ("disabled index (col)")) -> (element #1=w305:string[], element #2=w304:string[])  [unwired: 3 in]
        n175 = for {
          tunnel: w305 -> [w353] mode=indexing
          tunnel: w304 -> [w354] mode=indexing
          tunnel: [w352] -> w302 mode=indexing
          n176 = Empty String/Path?(string/path=w353) -> (empty?=w356:bool)
          n177 = Empty String/Path?(string/path=w354) -> (empty?=w357:bool)
          n178 = Or(x=w356, y=w357) -> (x .or. y?=w355:bool)
          n179 = case shown="False" w355 {
            tunnel: [w360 0.0] -> w352
            tunnel: w353 -> [w359 _]
            tunnel: w354 -> [w358 _]
            frame False {
              n180 = call "String to timestamp new.vi"("String Timestamp"=w359) -> ("Timestamp"=w362:timestamp)  [unwired: 10 in]
              n181 = call "String to timestamp new.vi"("String Timestamp"=w358) -> ("Timestamp"=w361:timestamp)  [unwired: 10 in]
              n182 = Max & Min(x=w362, y=w361) -> (max(x,y)=w366:timestamp, min(x,y)=w365:timestamp)
              n183 = To Double Precision Float(number=w366) -> (double precision float=w364:dbl)
              n184 = To Double Precision Float(number=w365) -> (double precision float=w363:dbl)
              n185 = Subtract(x=w364, y=w363) -> (x-y=w360:dbl)
            }
            frame True {
            }
          }
        }
        n186 = Add Array Elements(numeric array=w302) -> (sum=→"Q Duration Min" →"Duration Q":dbl)
        n187 = Merge Errors(w322, w321) -> (w320:errorcluster)
      }
      frame "5" {
        w413 = 0 ("index (row)")
        w416 = 0 ("index (row)")
        (unwired) "Select IS_ACTIVE  From STATION_1_LOG_HISTORY\nWhere LOG_ID='%s' \n\n"
        (unwired) "Select MAX(LOG_ID)  From STATION_1_LOG_HISTORY \n Where PLAN_DATE='%s' And BREAKDOWN_STK_HOLD_ID='5'\n\n"
        (unwired) "Select  BREAKDOWN_IN_TIME,BREAKDOWN_OUT_TIME,DATEDIFF (MINUTE,BREAKDOWN_IN_TIME,BREAKDOWN_OUT_TIME)\nFrom STATION_1_LOG_HISTORY\nWhere PLAN_DATE ='%s'  And BREAKDOWN_STK_HOLD_ID='5'\n\n"  # Select  BREAKDOWN_IN_TIME,BREAKDOWN_OUT_TIME,DATEDIFF (MINUTE,BREAKDOWN_IN_TIME,BREAKDOWN_OUT_TIME) From STATION_1_LOG_HISTORY Where PLAN_DATE ='%s'  And BREAKDOWN_STK_HOLD_ID='5'
        w429 = 0 ("index (row)")
        (unwired) "Select COUNT(LOG_ID)  From STATION_1_LOG_HISTORY \n Where PLAN_DATE='%s' And BREAKDOWN_STK_HOLD_ID='5'"  # Select COUNT(LOG_ID)  From STATION_1_LOG_HISTORY   Where PLAN_DATE='%s' And BREAKDOWN_STK_HOLD_ID='5'
        n188 = Concatenate Strings("Select IS_ACTIVE  From \n\n", w392, " Where LOG_ID='%s' \n\n") -> (w389:string)
        n189 = Concatenate Strings("Select MAX(LOG_ID)  From \n", w392, " Where PLAN_DATE='%s' And BREAKDOWN_STK_HOLD_ID='5'\n\n") -> (w397:string)
        n190 = global read "Current date.vi" "Current Date"() -> (w421:string)
        n191 = Concatenate Strings("Select COUNT(LOG_ID)  From \n", w392, " Where PLAN_DATE='%s' And BREAKDOWN_STK_HOLD_ID='5'\n\n") -> (w390:string)
        n192 = Concatenate Strings("Select  BREAKDOWN_IN_TIME,BREAKDOWN_OUT_TIME,DATEDIFF (MINUTE,BREAKDOWN_IN_TIME,BREAKDOWN_OUT_TIME)\nFROM " ("SQL query"), w392, " Where PLAN_DATE='%s' And BREAKDOWN_STK_HOLD_ID='5'\n\n") -> (w391:string)
        n193 = Format Into String(format string=w397, w421) -> (resulting string=w420:string)  [unwired: 2 in, 1 out]
        n194 = call "Execute query.vi"("error in (no error)"=w411, "String"=w420, "connection reference"=w410) -> ("error out"=w419:errorcluster, "Table"=w415:string[][], "connection reference 2"=w418:T1)  [unwired: 3 in, 3 out]
        n195 = global read "Current date.vi" "Current Date"() -> (w424:string)
        n196 = Index Array(array=w415, index (row)=w416, index (col)=w416) -> (element=w414:string)
        n197 = Format Into String(format string=w389, w414) -> (resulting string=w417:string)  [unwired: 2 in, 1 out]
        n198 = call "Execute query.vi"("error in (no error)"=w419, "String"=w417, "connection reference"=w418) -> ("error out"=w398:errorcluster, "Table"=w412:string[][], "connection reference 2"=w409:T1)  [unwired: 3 in, 3 out]
        n199 = Format Into String(format string=w390, w424) -> (resulting string=w431:string)  [unwired: 2 in, 1 out]
        n200 = Index Array(array=w412, index (row)=w413, index (col)=w413) -> (element=w408:string)
        n201 = call "Execute query.vi"("error in (no error)"=w398, "String"=w431, "connection reference"=w409) -> ("error out"=w427:errorcluster, "Table"=w430:string[][], "connection reference 2"=w426:T1)  [unwired: 3 in, 3 out]
        n202 = control-ref of="P Ack"() -> (w407:refnum<vi>)
        n203 = control-ref of="SS"() -> (w406:refnum<vi>)
        n204 = Index Array(array=w430, index (row)=w429, index (col)=w429) -> (element=w428:string)
        n205 = Decimal String To Number(string=w428) -> (number=→"P Counter" →"COUNT P":i32)  [unwired: 2 in, 1 out]
        n206 = case shown="\"3\", Default" w408 {
          tunnel: [w450 w457 w462] -> w403
          tunnel: w398 -> [w452 w454 w465]
          tunnel: w407 -> [_ w456 w464]
          tunnel: w406 -> [w451 w455 w461]
          frame "1" {
            n207 = property class="Bool"(reference=w451, error in=w452, "Colors [4]"=cluster{u32, u32}[] [{52224, 52224}]) -> (error out=w450:errorcluster)  [unwired: 1 out]
          }
          frame "3", Default {
            w458 = cluster{u32, u32}[] [{12369084, 12369084}] ("Colors [4]")
            n208 = property class="Bool"(reference=w455, error in=w454, "Colors [4]"=w458) -> (error out=w459:errorcluster)  [unwired: 1 out]
            n209 = property class="Bool"(reference=w456, error in=w459, "Colors [4]"=w458) -> (error out=w457:errorcluster)  [unwired: 1 out]
          }
          frame "2" {
            w460 = cluster{u32, u32}[] [{52224, 52224}] ("Colors [4]")
            n210 = property class="Bool"(reference=w464, error in=w465, "Colors [4]"=w460) -> (error out=w463:errorcluster)  [unwired: 1 out]
            n211 = property class="Bool"(reference=w461, error in=w463, "Colors [4]"=w460) -> (error out=w462:errorcluster)  [unwired: 1 out]
          }
        }
        n212 = Format Into String(format string=w391, w424) -> (resulting string=w423:string)  [unwired: 2 in, 1 out]
        n213 = call "Execute query.vi"("error in (no error)"=w427, "String"=w423, "connection reference"=w426) -> ("error out"=w405:errorcluster, "Table"=w385:string[][], "connection reference 2"=w425:T1)  [unwired: 3 in, 3 out]
        n214 = Index Array(array=w385, index (col) #1=0 ("disabled index (col)")) -> (element #1=w387:string[], element #2=w386:string[])  [unwired: 3 in]
        n215 = for {
          tunnel: w387 -> [w435] mode=indexing
          tunnel: w386 -> [w436] mode=indexing
          tunnel: [w434] -> w384 mode=indexing
          n216 = Empty String/Path?(string/path=w435) -> (empty?=w438:bool)
          n217 = Empty String/Path?(string/path=w436) -> (empty?=w439:bool)
          n218 = Or(x=w438, y=w439) -> (x .or. y?=w437:bool)
          n219 = case shown="False" w437 {
            tunnel: [w442 0.0] -> w434
            tunnel: w435 -> [w441 _]
            tunnel: w436 -> [w440 _]
            frame False {
              n220 = call "String to timestamp new.vi"("String Timestamp"=w441) -> ("Timestamp"=w444:timestamp)  [unwired: 10 in]
              n221 = call "String to timestamp new.vi"("String Timestamp"=w440) -> ("Timestamp"=w443:timestamp)  [unwired: 10 in]
              n222 = Max & Min(x=w444, y=w443) -> (max(x,y)=w448:timestamp, min(x,y)=w447:timestamp)
              n223 = To Double Precision Float(number=w448) -> (double precision float=w446:dbl)
              n224 = To Double Precision Float(number=w447) -> (double precision float=w445:dbl)
              n225 = Subtract(x=w446, y=w445) -> (x-y=w442:dbl)
            }
            frame True {
            }
          }
        }
        n226 = Add Array Elements(numeric array=w384) -> (sum=→"P Duration Min" →"Duration P":dbl)
        n227 = Merge Errors(w405, w403) -> (w404:errorcluster)
      }
    }
    n228 = Wait (ms)(milliseconds to wait=u32 100) -> ()  [unwired: 1 out]
    "Station Name" <- w36
  }
  n229 = property class="App"(error in=w30) -> (error out=w31:errorcluster, "App.Kind"=w32:T2)  [unwired: 1 in, 1 out]
  n230 = call <vilib>:"DB Tools Close Connection.vi"("connection reference"=w8) -> ("error out"=w7:errorcluster)  [unwired: 6 in]
  n231 = Unbundle By Name(w7) -> ()  [unwired: 1 out]
  n232 = case shown="\"Run Time System\"" w32 {
    tunnel: w31 -> [w467 w472]
    tunnel: [w466 w471] -> w10
    frame Default {
      n233 = disable-structure shown="Enabled" {
        disable-tunnel: w467 -> [w469 w470]
        disable-tunnel: [w468 w470] -> w466
        frame Disabled {
          n234 = invoke class="VI" method="FP.Close"(error in=w469) -> (error out=w468:errorcluster)  [unwired: 2 in, 2 out]
        }
        frame Enabled {
        }
      }
    }
    frame "Run Time System" {
      n235 = invoke class="VI" method="FP.Close"(error in=w472) -> (error out=w471:errorcluster)  [unwired: 2 in, 2 out]
    }
  }
  "error out" <- w10
